vi "Gen Cursor List.vi"(1 "Count in":i32, 2 "Settings in":T1={"Name"="Cursor 0", "Color"=16711680, "Style"=2, "Point Style"=13, "Name Visible"=FALSE, "Allow Drag"=TRUE, "Cursor Mode"=1, "Plot"=-1, "Index"=310, "Position"={"X"=50.1, "Y"=0.0}, "X Scale"=0, "Y Scale"=0, "Watch Plots"=[], "Watch All Plots"=FALSE, "Plot Area"=0, "Label Offset"={"X"=-0.00649752475247567, "Y"=6.211909771510491}}) -> (0 "CrsrLst Out":T2(array[cluster]))   [LabVIEW 2019]
doc: "Generates a lis to cursors based on inital settings and count."
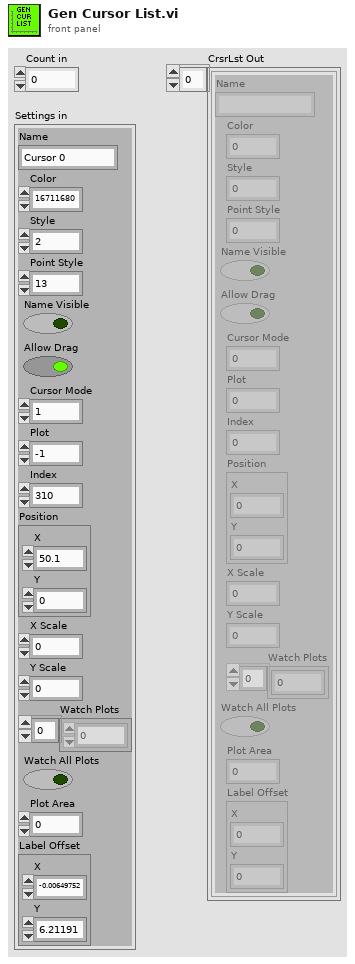
[diagram p1: front panel]
types:
  T1 = cluster{"Name":string, "Color":u32, "Style":i32, "Point Style":u8, "Name Visible":bool, "Allow Drag":bool, "Cursor Mode":u32, "Plot":i32, "Index":i32, "Position":cluster{"X":dbl, "Y":dbl}, "X Scale":u32, "Y Scale":u32, "Watch Plots":i32[], "Watch All Plots":bool, "Plot Area":i32, "Label Offset":cluster{"X":dbl, "Y":dbl}}
  T2 = cluster{"Name":string, "Color":u32, "Style":i32, "Point Style":u8, "Name Visible":bool, "Allow Drag":bool, "Cursor Mode":u32, "Plot":i32, "Index":i32, "Position":cluster{"X":dbl, "Y":dbl}, "X Scale":u32, "Y Scale":u32, "Watch Plots":i32[], "Watch All Plots":bool, "Plot Area":i32, "Label Offset":cluster{"X":dbl, "Y":dbl}}[]
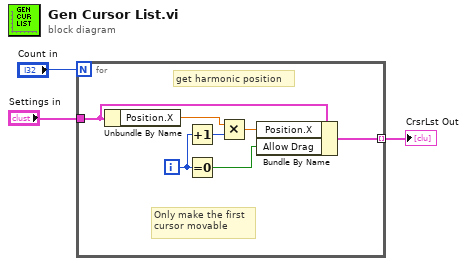
[diagram p0: block diagram]
diagram:
  n1 = for {
    N: "Count in" -> [_]
    tunnel: "Settings in" -> [w10]
    tunnel: [w6] -> w3 mode=indexing
    i -> [w5]
    # "get harmonic position"
    # "Only make the first\ncursor movable"
    n2 = Unbundle By Name(w10) -> ("Position.X"=w9:dbl)
    n3 = Increment(x=w5) -> (x+1=w8:i32)
    n4 = Equal To 0?(x=w5) -> (x = 0?=w4:bool)
    n5 = Multiply(x=w9, y=w8) -> (x*y=w7:dbl)
    n6 = Bundle By Name(cluster=w10, "Position.X"=w7, "Allow Drag"=w4) -> (w6:T1)
  }
  "CrsrLst Out" <- w3
